vi "SMO.vi"(0 "System no.":i32=1 min=1 max=4 step=1, 2 "Axes to set":string[](array[string]), 3 "Motor output":i32[](array[numeric]), 5 "error in":errorcluster) -> (14 "Controller error":bool, 19 "error out":errorcluster)   [LabVIEW 2020]
doc: "Sets the motor output directly and checks for error. Command will only be executed if channel is in servo-off mode (SVO.vi). \nCaution: In servo-off mode limit switches are not enabled! \nNo. of digits is the number of digits after the decimal point in the motor output value(s) that will be sent. Controller error is TRUE if selected system reports an error code which is not 0.\n\nAll systems: No. of digits is 0."
panel:
  # "Sets the motor output directly and checks for error. Command\nwill only be executed if channel is in servo-off mode (SVO.vi).\nCAUTION: In servo-off mode limit switches are not enabled!"
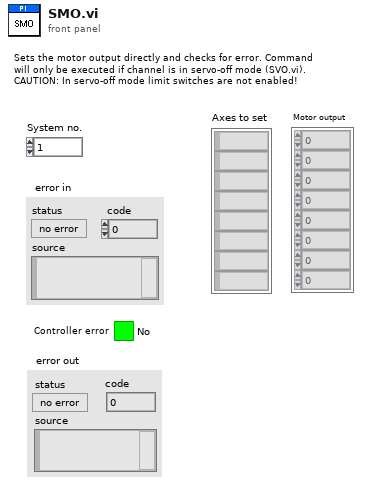
[diagram p1: front panel]
types:
  T1 = enum16{"Disable error check", "Force error check", "Use global settings"}
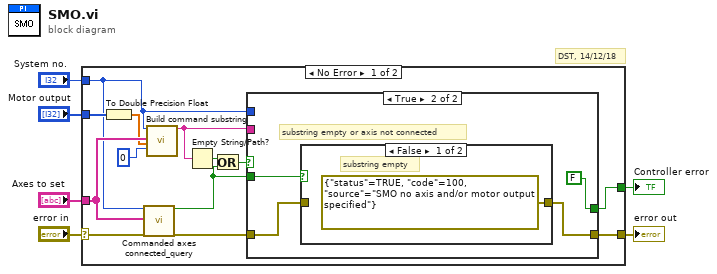
[diagram p0: block diagram]
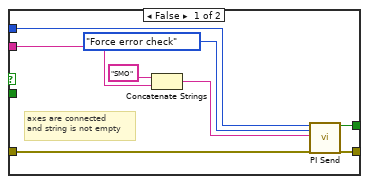
[diagram p2: hidden frame]
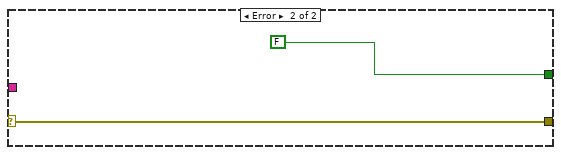
[diagram p4: hidden frame]
diagram:
  # "DST, 14/12/18"
  n1 = case shown="No Error" "error in" {
    selector: "error in" -> [w12 w34]
    tunnel: [w19 w34] -> w6
    tunnel: "Motor output" -> [w17 _]
    tunnel: "System no." -> [w8 _]
    tunnel: "Axes to set" -> [w15 _]
    tunnel: [w10 FALSE ("Controller error")] -> w1
    frame No Error {
      n2 = To Double Precision Float(number=w17) -> (double precision float=w7:dbl[])
      n3 = call "Commanded axes connected_query.vi"("System no."=w8, "Commanded axes"=w15, "error in"=w12) -> ("Controller error"=w11:bool, "error out"=w16:errorcluster)  [unwired: 1 in, 14 out]
      n4 = call "Build command substring.vi"("System no."=w8, "Affected axes"=w15, "Parameters"=w7, "No. of digits"=i16 0) -> ("Command substring"=w18:string)  [unwired: 3 in, 12 out]
      n5 = Empty String/Path?(string/path=w18) -> (empty?=w14:bool)
      n6 = Or(x=w14, y=w11) -> (x .or. y?=w13:bool)
      n7 = case shown="True" w13 {
        tunnel: w18 -> [w26 _]
        tunnel: [w22 w31] -> w19
        tunnel: w16 -> [w24 w29]
        tunnel: w11 -> [_ w30]
        tunnel: w8 -> [w23 _]
        tunnel: [w21 FALSE ("Controller error")] -> w10
        frame False {
          # "axes are connected\nand string is not empty"
          n8 = Concatenate Strings("SMO", w26) -> (w25:string)
          n9 = call "PI Send.vi"("System no."=w23, "Error check settings"=T1."Force error check", "String to send"=w25, "error in"=w24) -> ("Controller error"=w21:bool, "error out"=w22:errorcluster)  [unwired: 2 in, 12 out]
        }
        frame True {
          # "substring empty or axis not connected"
          n10 = case shown="False" w30 {
            tunnel: [errorcluster {"status"=TRUE, "code"=100, "source"="SMO no axis and/or motor output specified"} ("error out") w33] -> w31
            tunnel: w29 -> [_ w33]
            frame False {
              # "substring empty"
            }
            frame True {
              # "commanded axis\nnot connected"
            }
          }
        }
      }
    }
    frame Error {
    }
  }
  "error out" <- w6
  "Controller error" <- w1
